vi "Trim Whitespace+.vi"(0 "String":string, 1 "location (both)":T1 items=["both", "start of string", "end of string"]) -> (2 "Trimmed String":string)   [LabVIEW 2011, in "JSON Scalar.lvclass"]
doc: "Removes all ASCII white space (spaces, tabs, carriage returns, and linefeeds) from the beginning, end, or both ends of <B>string</B>. The Trim Whitespace VI does not remove double byte characters."
uses:
  JSON Scalar.lvclass
  <vilib>/Utility/error.llb/whitespace.ctl
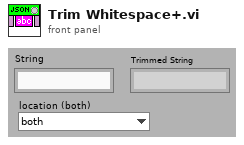
[diagram p1: front panel]
types:
  T1 = typedef "whitespace.ctl" = u16
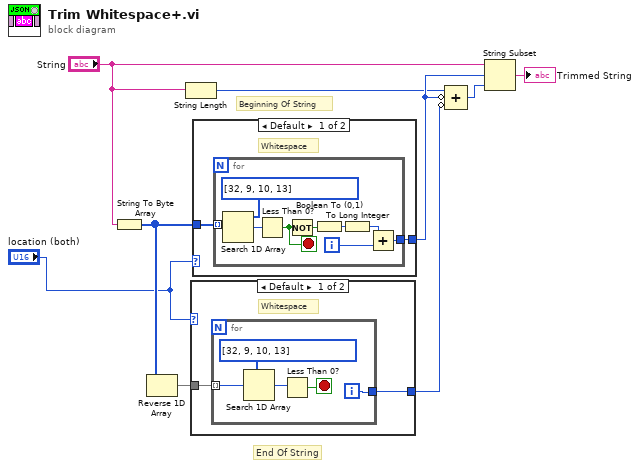
[diagram p0: block diagram]
diagram:
  # "End Of String"
  # "Beginning Of String"
  n1 = String To Byte Array(string="String") -> (unsigned byte array=w5:u8[])
  n2 = Reverse 1D Array(array=w5) -> (reversed array=w9:u8[])
  n3 = String Length(string="String") -> (length=w2:i32)
  n4 = case shown="Default" "location (both)" {
    tunnel: w9 -> [w11 _]
    tunnel: [w10 _] -> w6
    frame Default {
      # "Whitespace"
      n5 = for {
        tunnel: w11 -> [w15] mode=indexing
        tunnel: [w16] -> w10
        i -> [w16]
        stop <- w12 stop-if-true
        n6 = Search 1D Array(1D array=u8[] [32, 9, 10, 13], element=w15) -> (index of element=w13:i32)  [unwired: 1 in]
        n7 = Less Than 0?(x=w13) -> (x < 0?=w12:bool)
      }
    }
    frame 1 {
    }
  }
  n8 = case shown="Default" "location (both)" {
    tunnel: w5 -> [w18 _]
    tunnel: [w17 _] -> w4
    frame Default {
      # "Whitespace"
      n9 = for {
        tunnel: w18 -> [w26] mode=indexing
        tunnel: [w22] -> w17
        i -> [w27]
        stop <- w23 stop-if-true
        n10 = Search 1D Array(1D array=u8[] [32, 9, 10, 13], element=w26) -> (index of element=w24:i32)  [unwired: 1 in]
        n11 = Less Than 0?(x=w24) -> (x < 0?=w23:bool)
        n12 = Not(x=w23) -> (.not. x?=w20:bool)
        n13 = Boolean To (0,1)(Boolean=w20) -> (0, 1=w21:i16)
        n14 = To Long Integer(number=w21) -> (32bit integer=w19:i32)
        n15 = Add(x=w19, y=w27) -> (x+y=w22:i32)
      }
    }
    frame 2 {
    }
  }
  n16 = Compound Arithmetic op=ADD(w2, invert w4, invert w6) -> (w3:i32)
  n17 = String Subset(string="String", offset (0)=w4, length (rest)=w3) -> (substring=→"Trimmed String":string)
